vi "user initialization.vi"(8 "error in":errorcluster, 10 "configuration in":refnum<class "control module configuration.lvclass">, 11 "fixed channel runtime in":refnum<class "AppStateMachine runtime.lvclass">) -> (0 "error out":errorcluster, 3 "fixed channel runtime out":refnum<class "AppStateMachine runtime.lvclass">)   [LabVIEW 2017, in "AppStateMachine runtime.lvclass"]
uses:
  AppStateMachine runtime.lvclass
  <vilib>/NI/DCAF/Tag Editor Core/control module/configuration/control module configuration.lvclass
  FPGA_FGV_action.ctl
  <vilib>/userdefined/High Color/nirio_resource_hc.ctl
  State.ctl
  AppStateMachine runtime.lvclass/AppStateMachine runtime.ctl
  <vilib>/NI/DCAF/Tag Editor Core/control module/runtime/control module runtime.lvclass
  <vilib>/NI/NI JSONRPC Server Framework/Classes/Server/JSONRPC Server.lvclass
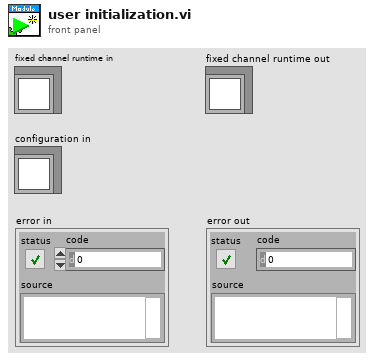
[diagram p1: front panel]
types:
  T1 = typedef "AppStateMachine runtime.lvclass/State.ctl" = enum16{"Initialize", "Idle", "Starting", "Running", "Stopping"}
  T2 = typedef "nirio_resource_hc.ctl" = tag
  T3 = typedef "FPGA_FGV_action.ctl" = enum16{"get FPGA", "set FPGA", "Close"}
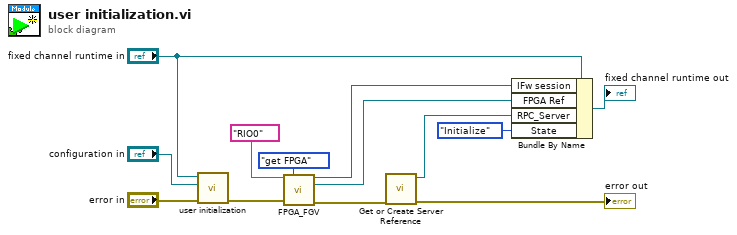
[diagram p0: block diagram]
diagram:
  n1 = call-parent "user initialization.vi"("error in"="error in", "configuration in"="configuration in", "fixed channel runtime in"="fixed channel runtime in") -> ("error out"=w11:errorcluster)  [unwired: 7 in, 1 out]
  n2 = call "FPGA_FGV.vi"("RIO resource"=T2 "RIO0", "Action"=FPGA_FGV_action."get FPGA", "error in"=w11) -> ("session out"=w8:refnum<class "niInstr FIFO Register Bus v1 Host.lvclass">, "bitfile"=w7:refnum<k20>, "error out"=w4:errorcluster)  [unwired: 10 in]
  n3 = call <vilib>:"Get or Create Server Reference.vi"("error in (no error)"=w4) -> ("error out"=→"error out":errorcluster, "Server Out"=w2:refnum<class "JSONRPC Server.lvclass">)  [unwired: 9 in]
  n4 = Bundle By Name(cluster="fixed channel runtime in", "IFw session"=w8, "FPGA Ref"=w7, "RPC_Server"=w2, "State"=State."Initialize") -> (→"fixed channel runtime out":refnum<class "AppStateMachine runtime.lvclass">)
